vi "reql_table_drop.vi"(6 "ms timeout (0:default)":i32, 7 "db name":string, 8 "error in (no error)":errorcluster, 10 "table name":string, 11 "rethinkdb in":refnum<class "RethinkDB.lvclass">) -> (0 "error out":errorcluster, 2 "table exists?":bool, 3 "rethinkdb out":refnum<class "RethinkDB.lvclass">, 4 "response":variant)   [LabVIEW 2017, in "rethinkdb.lvlib"]
uses:
  rethinkdb.lvlib
  RethinkDB.lvclass
  ql2_term.ctl
  ql2_query.ctl
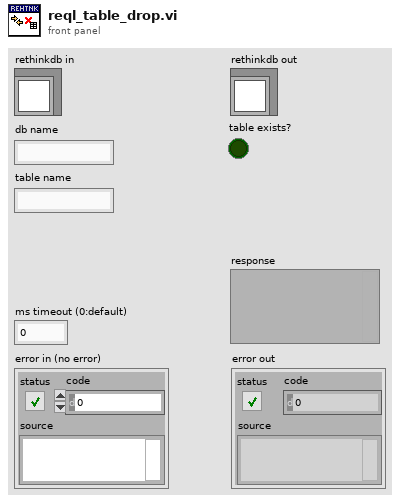
[diagram p1: front panel]
types:
  T1 = typedef "rethinkdb.lvlib/ql2_query.ctl" = enum8{"START", "CONTINUE", "STOP", "NOREPLY_WAIT", "SERVER_INFO", "invalid"}
  T2 = typedef "rethinkdb.lvlib/ql2_term.ctl" = enum8{"ADD", "AND", "APPEND", "APRIL", "ARGS", "ASC", "AUGUST", "AVG", "BETWEEN", "BETWEEN_DEPRECATED", "BINARY", "BIT_AND", "BIT_NOT", "BIT_OR", "BIT_SAL", "BIT_SAR", "BIT_XOR", "BRACKET", "BRANCH", "CEIL", "CHANGES", "CHANGE_AT", "CIRCLE", "COERCE_TO", "CONCAT_MAP", "CONFIG", "CONTAINS", "COUNT", "DATE", "DATUM", "DAY", "DAY_OF_WEEK", "DAY_OF_YEAR", "DB", "DB_CREATE", "DB_DROP", "DB_LIST", "DECEMBER", "DEFAULT", "DELETE", "DELETE_AT", "DESC", "DIFFERENCE", "DISTANCE", "DISTINCT", "DIV", "DOWNCASE", "DURING", "EPOCH_TIME", "EQ", "EQ_JOIN", "ERROR", "FEBRUARY", "FILL", "FILTER", "FLOOR", "FOLD", "FOR_EACH", "FRIDAY", "FUNC", "FUNCALL", "GE", "GEOJSON", "GET", "GET_ALL", "GET_FIELD", "GET_INTERSECTING", "GET_NEAREST", "GET_WRITE_HOOK", "GRANT", "GROUP", "GT", "HAS_FIELDS", "HOURS", "HTTP", "IMPLICIT_VAR", "INCLUDES", "INDEX_CREATE", "INDEX_DROP", "INDEX_LIST", "INDEX_RENAME", "INDEX_STATUS", "INDEX_WAIT", "INFO", "INNER_JOIN", "INSERT", "INSERT_AT", "INTERSECTS", "IN_TIMEZONE", "ISO8601", "IS_EMPTY", "JANUARY", "JAVASCRIPT", "JSON", "JULY", "JUNE", "KEYS", "LE", "LIMIT", "LINE", "LITERAL", "LT", "MAKE_ARRAY", "MAKE_OBJ", "MAP", "MARCH", "MATCH", "MAX", "MAXVAL", "MAY", "MERGE", "MIN", "MINUTES", "MINVAL", "MOD", "MONDAY", "MONTH", "MUL", "NE", "NOT", "NOVEMBER", "NOW", "NTH", "OBJECT", "OCTOBER", "OFFSETS_OF", "OR", "ORDER_BY", "OUTER_JOIN", "PLUCK", "POINT", "POLYGON", "POLYGON_SUB", "PREPEND", "RANDOM", "RANGE", "REBALANCE", "RECONFIGURE", "REDUCE", "REPLACE", "ROUND", "SAMPLE", "SATURDAY", "SECONDS", "SEPTEMBER", "SET_DIFFERENCE", "SET_INSERT", "SET_INTERSECTION", "SET_UNION", "SET_WRITE_HOOK", "SKIP", "SLICE", "SPLICE_AT", "SPLIT", "STATUS", "SUB", "SUM", "SUNDAY", "SYNC", "TABLE", "TABLE_CREATE", "TABLE_DROP", "TABLE_LIST", "THURSDAY", "TIME", "TIMEZONE", "TIME_OF_DAY", "TO_EPOCH_TIME", "TO_GEOJSON", "TO_ISO8601", "TO_JSON_STRING", "TUESDAY", "TYPE_OF", "UNGROUP", "UNION", "UPCASE", "UPDATE", "UUID", "VALUES", "VAR", "WAIT", "WEDNESDAY", "WITHOUT", "WITH_FIELDS", "YEAR", "ZIP", "invalid"}
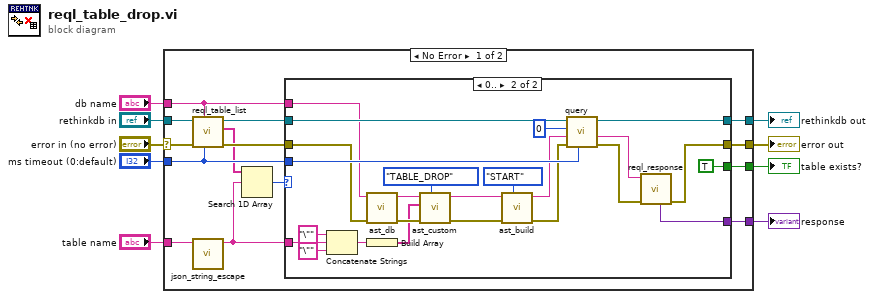
[diagram p0: block diagram]
diagram:
  n1 = case shown="No Error" "error in (no error)" {
    selector: "error in (no error)" -> [w20 w51]
    tunnel: "rethinkdb in" -> [w18 w50]
    tunnel: [w23 w50] -> w7
    tunnel: "ms timeout (0:default)" -> [w16 _]
    tunnel: [w22 w51] -> w5
    tunnel: "db name" -> [w15 _]
    tunnel: [w21 _] -> w3
    tunnel: "table name" -> [w14 _]
    tunnel: [w10 _] -> w1
    frame No Error {
      n2 = call "reql_table_list.vi"("ms timeout (0:default)"=w16, "db name"=w15, "error in (no error)"=w20, "rethinkdb in"=w18) -> ("error out"=w19:errorcluster, "table list"=w13:string[], "rethinkdb out"=w17:refnum<class "RethinkDB.lvclass">)  [unwired: 4 in, 1 out]
      n3 = call "json_string_escape.vi"("string"=w14) -> ("escaped string"=w12:string)  [unwired: 10 in]
      n4 = Search 1D Array(1D array=w13, element=w12) -> (index of element=w11:i32)  [unwired: 1 in]
      n5 = case shown="0.." w11 {
        tunnel: [w24 w49] -> w23
        tunnel: [w25 w45] -> w22
        tunnel: [_ w37] -> w21
        tunnel: w19 -> [w25 w33]
        tunnel: w17 -> [w24 w44]
        tunnel: w16 -> [_ w43]
        tunnel: w15 -> [_ w34]
        tunnel: w12 -> [_ w40]
        tunnel: [_ TRUE] -> w10
        frame ..-1 {
        }
        frame 0.. {
          n6 = Concatenate Strings("\"" ("string"), w40, "\"" ("string")) -> (w39:string)
          n7 = call "ast_db.vi"("error in (no error)"=w33, "db name"=w34) -> ("error out"=w32:errorcluster, "r.db"=w30:string)  [unwired: 8 in]
          n8 = Build Array(w39) -> (w26:string[])
          n9 = call "ast_custom.vi"("term_type"=ql2_term."TABLE_DROP", "error in (no error)"=w32, "args"=w26, "arg0"=w30) -> ("error out"=w29:errorcluster, "r"=w28:string)  [unwired: 6 in]
          n10 = call "ast_build.vi"("query_type"=ql2_query."START", "error in (no error)"=w29, "term"=w28) -> ("error out"=w27:errorcluster, "query"=w35:string)  [unwired: 7 in]
          n11 = call "query.vi"("ms timeout (0:default)"=w43, "error in (no error)"=w27, "query"=w35, "token in (random)"=u64 0, "rethinkdb in"=w44) -> ("error out"=w47:errorcluster, "response"=w46:string, "rethinkdb out"=w49:refnum<class "RethinkDB.lvclass">)  [unwired: 3 in, 1 out]
          n12 = call "reql_response.vi"("error in (no error)"=w47, "response"=w46) -> ("error out"=w45:errorcluster, "response"=w37:variant)  [unwired: 7 in, 1 out]
        }
      }
    }
    frame Error {
    }
  }
  "error out" <- w5
  "rethinkdb out" <- w7
  "response" <- w3
  "table exists?" <- w1
